vi "Get_IPAddress.vi"(8 "error in (no error)":errorcluster, 11 ".NET Reference in":refnum<k24>) -> (0 "error out":errorcluster, 1 "address":string, 3 "Reference out":refnum<k24>)   [LabVIEW 2017]
uses:
  C:/Users/Ssantec_Test/Documents/Instrument_DLL_Sample_Labview_20220902_Ver1.2.2/DLL/x86/InstrumentDLL.dll
  DLL/x86/InstrumentDLL.dll
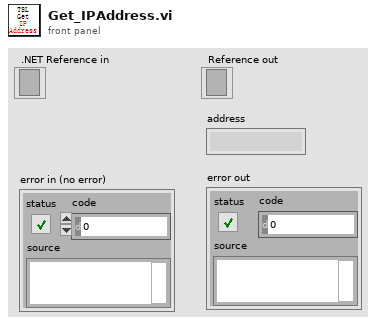
[diagram p1: front panel]
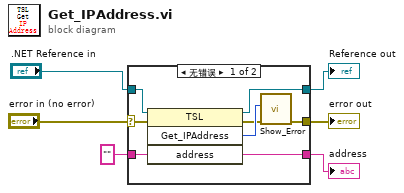
[diagram p0: block diagram]
diagram:
  n1 = case shown="无错误" "error in (no error)" {
    selector: "error in (no error)" -> [w7 w17]
    tunnel: ".NET Reference in" -> [w14 w15]
    tunnel: [w13 w15] -> w5
    tunnel: [w8 w17] -> w4
    tunnel: [w12 w16] -> w3
    tunnel: "" ("address") -> [w11 w16]
    frame No Error {
      n2 = invoke on="调用节点" class="TSL" method="Get_IPAddress"(reference=w14, error in=w7, "address"=w11) -> (reference out=w13:refnum<k24>, error out=w9:errorcluster, "Get_IPAddress"=w10:i32, "address"=w12:string)  [unwired: 1 in]
      n3 = call "Show_Error.vi"("error in (no error)"=w9, "Error"=w10) -> ("error out"=w8:errorcluster)  [unwired: 9 in]
    }
    frame Error {
    }
  }
  "Reference out" <- w5
  "error out" <- w4
  "address" <- w3
